vi "单IP测试.vi"(0 "服务端地址":string, 1 "远程端口/服务名称":u16, 3 "本地端口":u16, 8 "连接设置":bool, 11 "模拟数组":u16[](array[numeric]), 16 "06记录":string[][](table), 19 "16记录":string[][](table)) -> (9 "本机ip":string, 12 "接收数据":string, 13 "实时数据":string, 14 "03记录（去重）":string[][](table))   [LabVIEW 2019]
panel:
  out "下发报文":string
  out "格式转换-测试":string
  out "寄存器地址":u16
  out "功能码":u8
  out "从机地址":u8
  in  "停止":bool
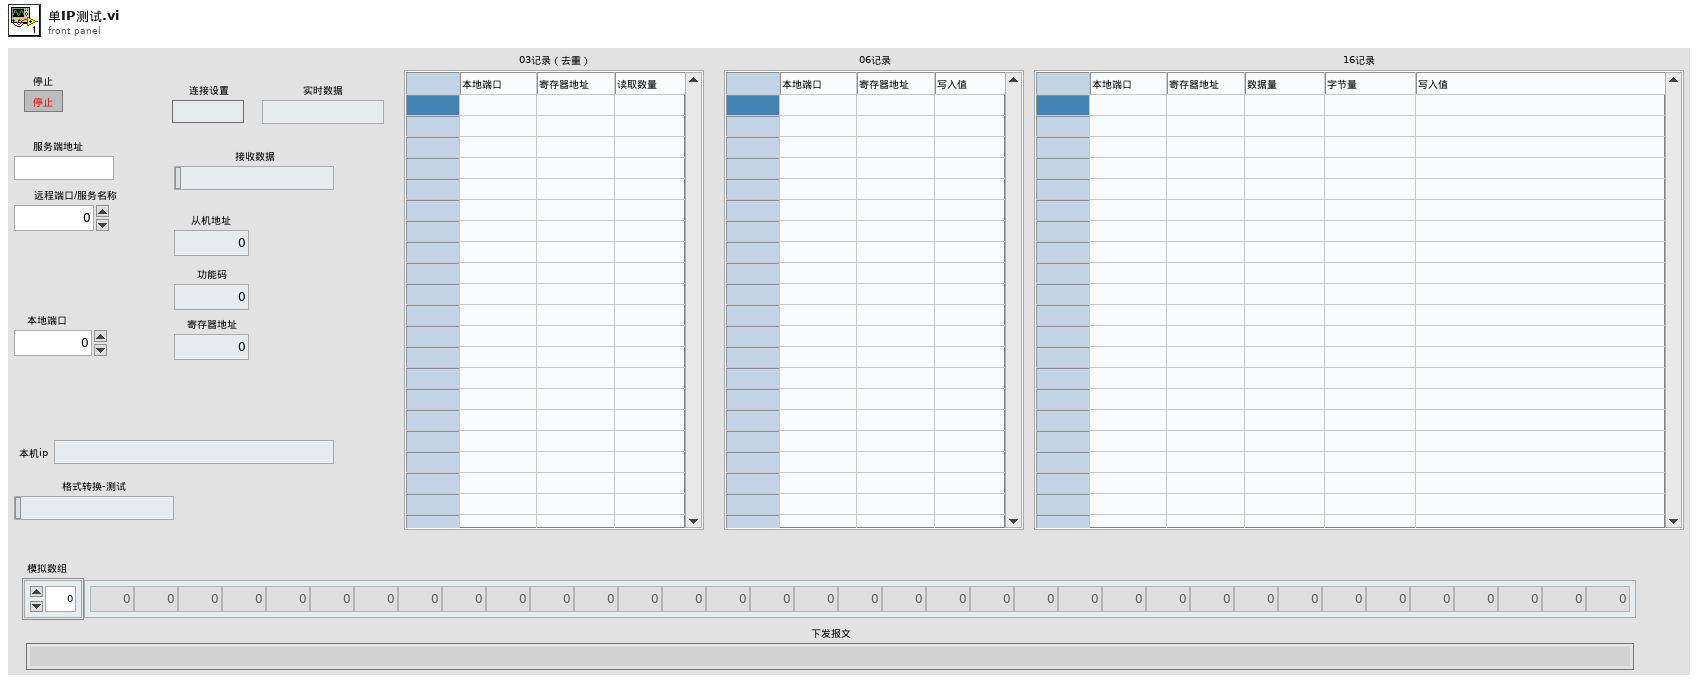
[diagram p1: front panel]
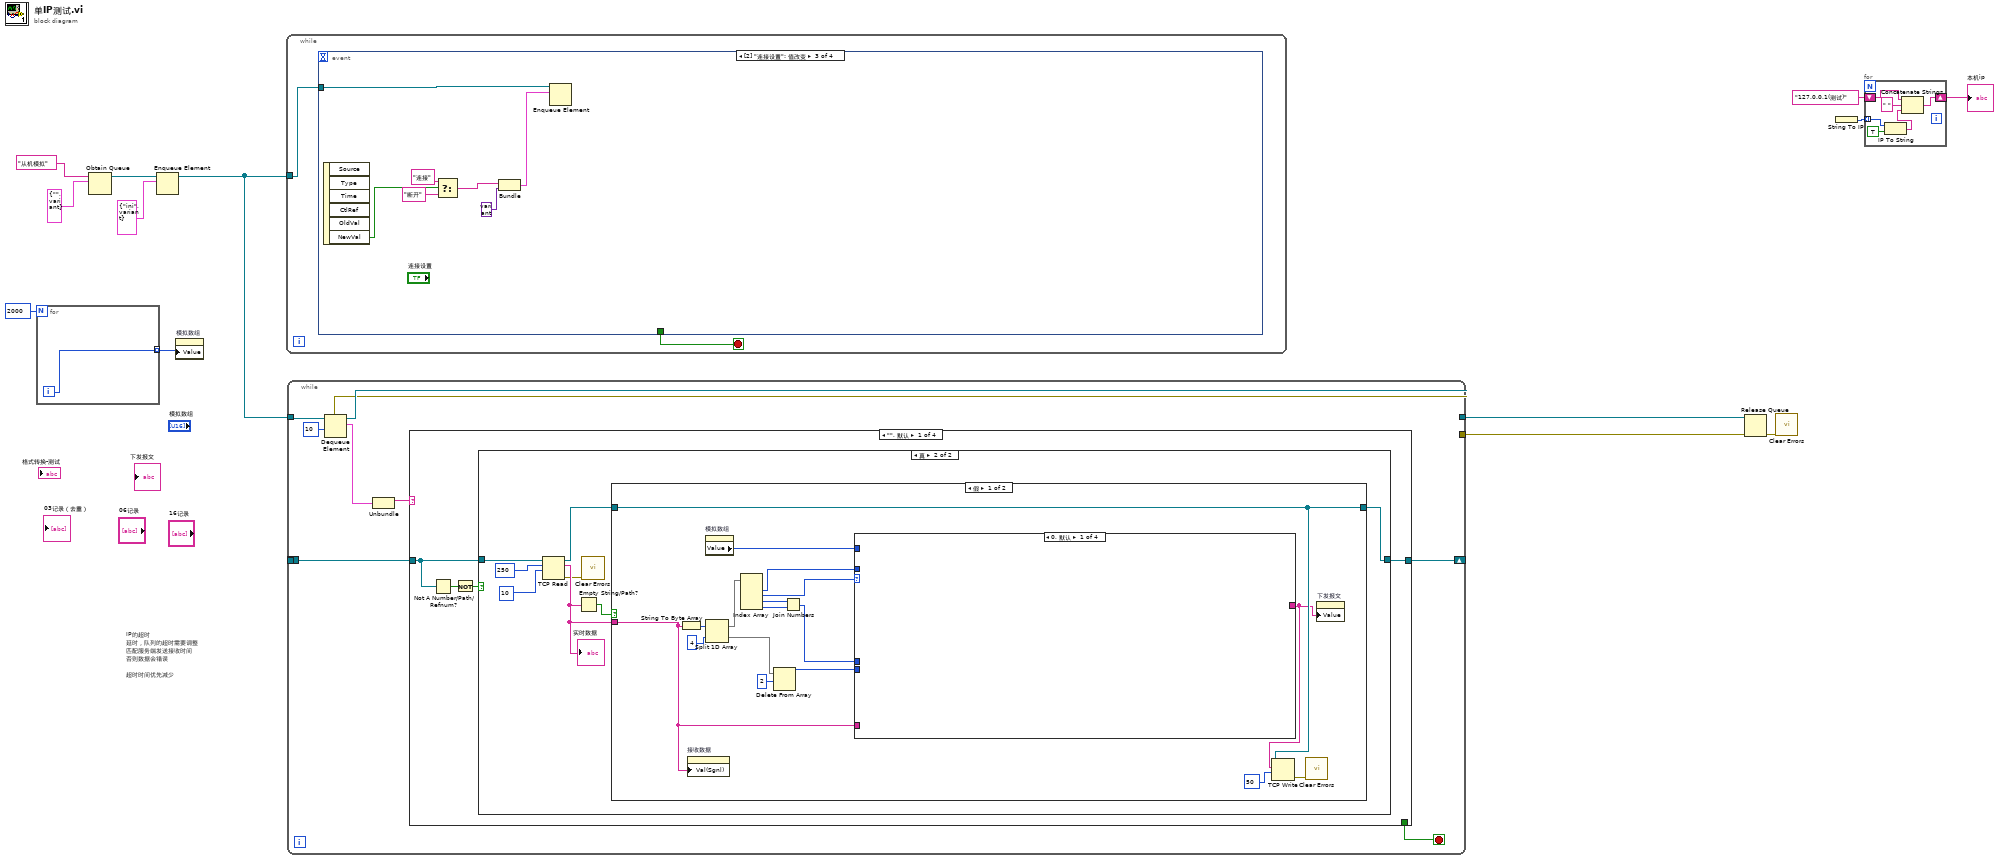
[diagram p0: block diagram]
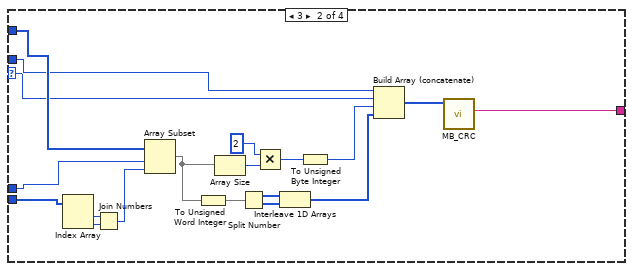
[diagram p3: hidden frame]
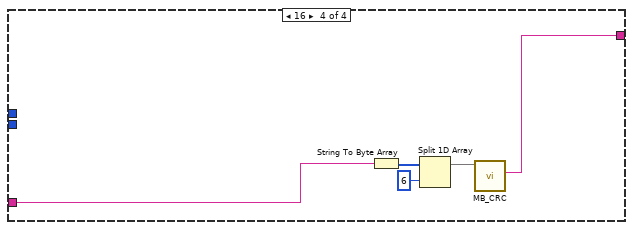
[diagram p5: hidden frame]
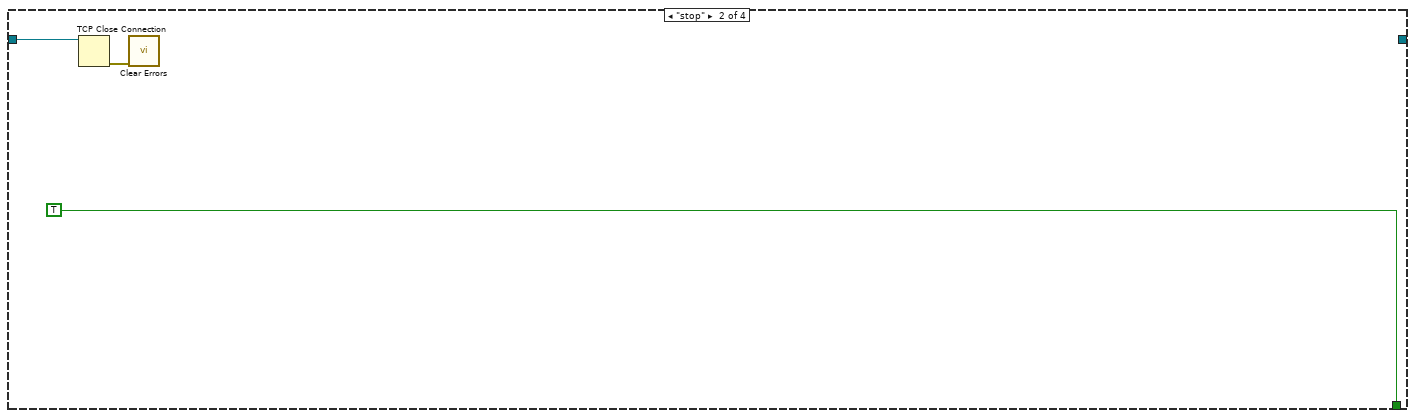
[diagram p7: hidden frame]
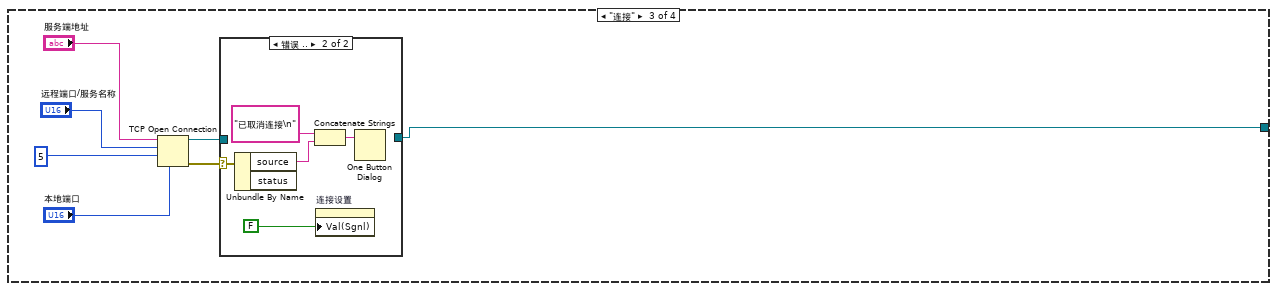
[diagram p8: hidden frame]
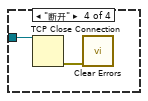
[diagram p10: hidden frame]
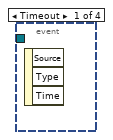
[diagram p11: hidden frame]
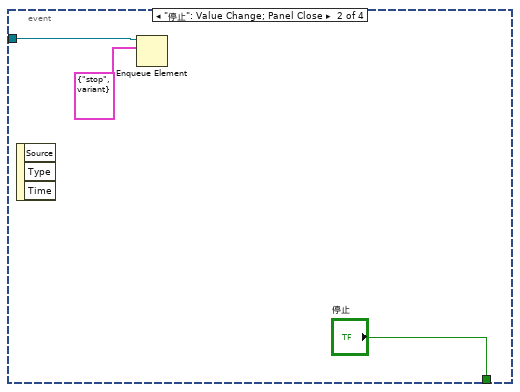
[diagram p12: hidden frame]
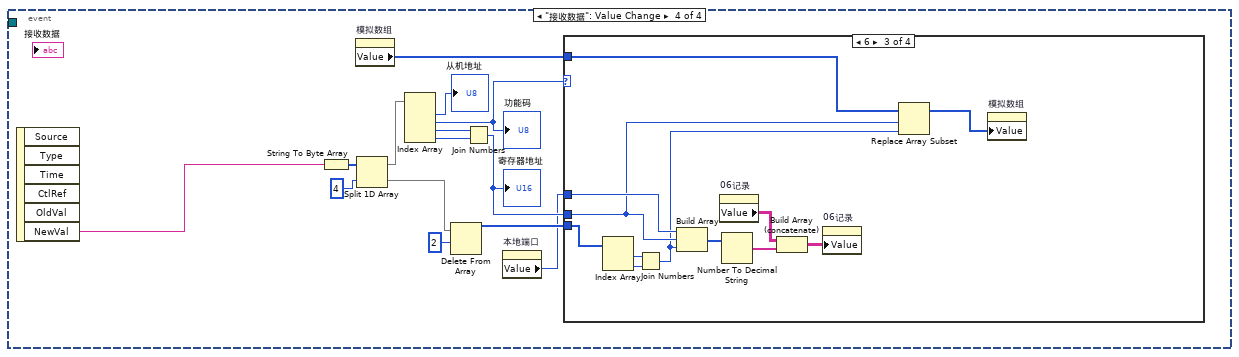
[diagram p13: hidden frame]
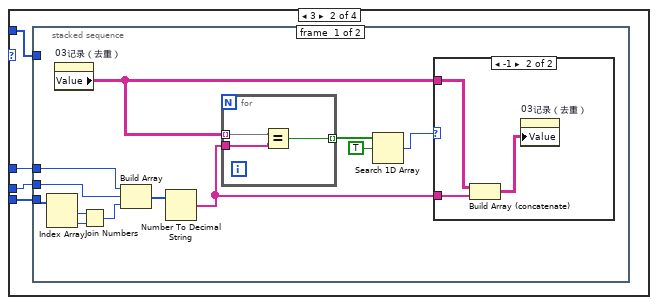
[diagram p15: hidden frame]
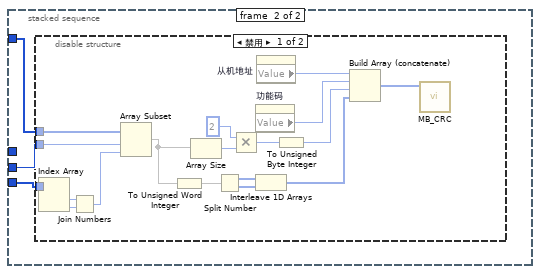
[diagram p17: hidden frame]
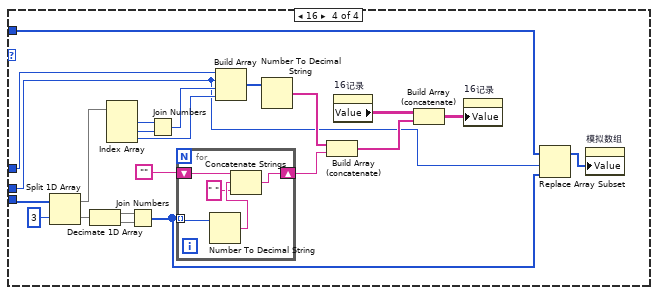
[diagram p19: hidden frame]
diagram:
  # "IP的超时\n延时，队列的超时需要调整\n匹配服务端发送接收时间\n否则数据会错误\n\n超时时间优先减少"
  n1 = for {
    N: 2000 -> [_]
    tunnel: [w14] -> w1 mode=indexing
    i -> [w14]
  }
  n2 = Obtain Queue(name (unnamed)="从机模拟" ("名称（未命名）"), element data type=cluster{string, variant} {"", variant}) -> (queue out=w8:refnum<queue>)  [unwired: 3 in, 2 out]
  n3 = Enqueue Element(queue=w8, element=cluster{string, variant} {"ini", variant} ("元素")) -> (queue out=w6:refnum<queue>)  [unwired: 2 in, 2 out]
  n4 = property on="模拟数组" class="Arr (严格)"("Value"=w1) -> ()  [unwired: 2 in, 2 out]
  n5 = while {
    tunnel: w6 -> [w16]
    stop <- w15 stop-if-true
    n6 = event shown="[2] \"连接设置\": 值改变" {
      selector: _ -> [_ _ _ _]
      dyn-events: _ -> [_ _ _ _]
      timeout: _ -> [_ _ _ _]
      tunnel: [_ "停止" _ _] -> w15
      tunnel: w16 -> [_ w18 w26 _]
      event Timeout {
        n7 = event-data() -> ()  [unwired: 1 in, 3 out]
      }
      event "停止": Value Change; Panel Close {
        n8 = event-data() -> ()  [unwired: 1 in, 3 out]
        n9 = Enqueue Element(queue=w18, element=cluster{string, variant} {"stop", variant} ("元素")) -> ()  [unwired: 2 in, 3 out]
      }
      event "连接设置": Value Change {
        n10 = event-data() -> ("NewVal"=w25:bool)  [unwired: 1 in, 5 out]
        n11 = Select(t="连接", s=w25, f="断开") -> (s? t:f=w23:string)
        n12 = Bundle("f"=w23, variant) -> (w22:cluster{"f":string, variant})  [unwired: 1 in]
        n13 = Enqueue Element(queue=w26, element=w22) -> ()  [unwired: 2 in, 3 out]
      }
      event "接收数据": Value Change {
        n14 = event-data() -> ("NewVal"=w32:string)  [unwired: 1 in, 5 out]
        n15 = String To Byte Array(string=w32) -> (unsigned byte array=w35:u8[])
        n16 = property on="模拟数组" class="Arr (严格)"() -> ("Value"=w27:u16[])  [unwired: 2 in, 2 out]
        n17 = Split 1D Array(array=w35, index=4 ("索引")) -> (first subarray=w36:u8[], second subarray=w40:u8[])
        n18 = Index Array(array=w36) -> (element #1=→"从机地址":u8, element #2=w31:u8, element #3=w38:u8, element #4=w39:u8)  [unwired: 4 in]
        "功能码" <- w31
        n19 = Delete From Array(array=w40, length=2 ("长度")) -> (array with subset deleted=w30:u8[])  [unwired: 1 in, 1 out]
        n20 = Join Numbers(hi=w38, lo=w39) -> ((hi.lo)=w29:u16)
        "寄存器地址" <- w29
        n21 = property on="本地端口" class="DigNum (严格)"() -> ("Value"=w28:u16)  [unwired: 2 in, 2 out]
        n22 = case shown="6" w31 {
          tunnel: w30 -> [_ w43 w91 w116]
          tunnel: w29 -> [_ w44 w86 w98]
          tunnel: w28 -> [_ w42 w90 w117]
          tunnel: w27 -> [_ w41 w87 w99]
          frame 0, Default {
          }
          frame 3 {
            n23 = stacked-sequence {
              tunnel: w44 -> [w56 w64]
              tunnel: w43 -> [w55 w63]
              tunnel: w42 -> [w45 _]
              tunnel: w41 -> [_ w65]
              frame #0 {
                n24 = Index Array(array=w55) -> (element #1=w47:u8, element #2=w48:u8)  [unwired: 2 in]
                n25 = property on="03记录（去重）" class="Tbl (严格)"() -> ("Value"=w49:string[][])  [unwired: 2 in, 2 out]
                n26 = Join Numbers(hi=w47, lo=w48) -> ((hi.lo)=w46:u16)
                n27 = Build Array(w45, w56, w46) -> (w54:u16[])
                n28 = Number To Decimal String(number=w54) -> (decimal integer string=w50:string[])  [unwired: 1 in]
                n29 = for {
                  tunnel: w50 -> [w61]
                  tunnel: w49 -> [w62] mode=indexing
                  tunnel: [w60] -> w53 mode=indexing
                  n30 = Equal?(x=w62, y=w61) -> (x = y?=w60:bool)
                }
                n31 = Search 1D Array(1D array=w53, element=TRUE ("元素")) -> (index of element=w51:i32)  [unwired: 1 in]
                n32 = case shown="-1" w51 {
                  tunnel: w50 -> [_ w59]
                  tunnel: w49 -> [_ w58]
                  frame 0, Default {
                  }
                  frame -1 {
                    n33 = Build Array (concatenate)(w58, w59) -> (w57:string[][])
                    n34 = property on="03记录（去重）" class="Tbl (严格)"("Value"=w57) -> ()  [unwired: 2 in, 2 out]
                  }
                }
              }
              frame #1 {
                n35 = disable-structure shown="禁用" {
                  disable-tunnel: w65 -> [w83 _]
                  disable-tunnel: w64 -> [w82 _]
                  disable-tunnel: w63 -> [w81 _]
                  frame Disabled {
                    n36 = Index Array(array=w81) -> (element #1=w77:u8, element #2=w78:u8)  [unwired: 2 in]
                    n37 = Join Numbers(hi=w77, lo=w78) -> ((hi.lo)=w76:u16)
                    n38 = Array Subset(array=w83, index=w82, length=w76) -> (w70:u16[])
                    n39 = To Unsigned Word Integer(number=w70) -> (unsigned 16bit integer=w69:u16[])
                    n40 = Array Size(array=w70) -> (size(s)=w75:i32)
                    n41 = Split Number(x=w69) -> (hi(x)=w68:u8[], lo(x)=w67:u8[])
                    n42 = Multiply(x=2, y=w75) -> (x*y=w73:i32)
                    n43 = property on="功能码" class="DigNum (严格)"() -> ("Value"=w79:u8)  [unwired: 2 in, 2 out]
                    n44 = Interleave 1D Arrays(w68, w67) -> (w66:u8[])
                    n45 = property on="从机地址" class="DigNum (严格)"() -> ("Value"=w80:u8)  [unwired: 2 in, 2 out]
                    n46 = To Unsigned Byte Integer(number=w73) -> (unsigned 8bit integer=w72:u8)
                    n47 = Build Array (concatenate)(w80, w79, w72, w66) -> (w71:u8[])
                    n48 = call "MB_CRC.vi"("无校验U8数组"=w71) -> ()  [unwired: 6 in, 2 out]
                  }
                  frame Enabled {
                  }
                }
              }
            }
          }
          frame 6 {
            n49 = Index Array(array=w91) -> (element #1=w92:u8, element #2=w93:u8)  [unwired: 2 in]
            n50 = Join Numbers(hi=w92, lo=w93) -> ((hi.lo)=w85:u16)
            n51 = Build Array(w90, w86, w85) -> (w95:u16[])
            n52 = property on="06记录" class="Tbl (严格)"() -> ("Value"=w89:string[][])  [unwired: 2 in, 2 out]
            n53 = Number To Decimal String(number=w95) -> (decimal integer string=w94:string[])  [unwired: 1 in]
            n54 = Build Array (concatenate)(w89, w94) -> (w88:string[][])
            n55 = property on="06记录" class="Tbl (严格)"("Value"=w88) -> ()  [unwired: 2 in, 2 out]
            n56 = Replace Array Subset(array=w87, new element=w85, index=w86) -> (w84:u16[])
            n57 = property on="模拟数组" class="Arr (严格)"("Value"=w84) -> ()  [unwired: 2 in, 2 out]
          }
          frame 16 {
            n58 = Split 1D Array(array=w116, index=3 ("索引")) -> (first subarray=w114:u8[], second subarray=w108:u8[])
            n59 = Decimate 1D Array(w108) -> (w107:u8[], w106:u8[])
            n60 = Index Array(array=w114) -> (element #1=w113:u8, element #2=w112:u8, element #3=w110:u8)  [unwired: 3 in]
            n61 = Join Numbers(hi=w107, lo=w106) -> ((hi.lo)=w97:u16[])
            n62 = Join Numbers(hi=w113, lo=w112) -> ((hi.lo)=w111:u16)
            n63 = for {
              tunnel: w97 -> [w122] mode=indexing
              shift-right: [w119] -> w103
              shift-left: "" -> [w118]
              n64 = Number To Decimal String(number=w122) -> (decimal integer string=w121:string)  [unwired: 1 in]
              n65 = Concatenate Strings(w118, w121, " " ("字符串")) -> (w119:string)
            }
            n66 = Build Array(w117, w98, w111, w110) -> (w109:u16[])
            n67 = Number To Decimal String(number=w109) -> (decimal integer string=w104:string[])  [unwired: 1 in]
            n68 = Build Array (concatenate)(w104, w103) -> (w101:string[])
            n69 = property on="16记录" class="Tbl (严格)"() -> ("Value"=w102:string[][])  [unwired: 2 in, 2 out]
            n70 = Build Array (concatenate)(w102, w101) -> (w100:string[][])
            n71 = property on="16记录" class="Tbl (严格)"("Value"=w100) -> ()  [unwired: 2 in, 2 out]
            n72 = Replace Array Subset(array=w99, new element=w97, index=w98) -> (w96:u16[])
            n73 = property on="模拟数组" class="Arr (严格)"("Value"=w96) -> ()  [unwired: 2 in, 2 out]
          }
        }
      }
    }
  }
  n74 = while {
    tunnel: w6 -> [w131]
    tunnel: [w128] -> w5
    tunnel: [w125] -> w4
    tunnel: [w123] -> _
    shift-right: [w124] -> _
    shift-left: _ -> [w123]
    stop <- w126 stop-if-true
    n75 = Dequeue Element(queue=w131, timeout in ms (-1)=10 ("超时毫秒(-1)")) -> (queue out=w128:refnum<queue>, element=w129:cluster{string, variant}, error out=w125:errorcluster)  [unwired: 1 in, 1 out]
    n76 = Unbundle(w129) -> (w127:string)  [unwired: 1 out]
    n77 = case shown="\"\", 默认" w127 {
      tunnel: [_ TRUE _ _] -> w126
      tunnel: w123 -> [w133 w188 _ w204]
      tunnel: [w132 _ w192 _] -> w124
      frame "", Default {
        n78 = Not A Number/Path/Refnum?(number/path/refnum=w133) -> (NaN/Path/Refnum?=w134:bool)
        n79 = Not(x=w134) -> (.not. x?=w135:bool)
        n80 = case shown="真" w135 {
          tunnel: w133 -> [w136 w144]
          tunnel: [w136 w137] -> w132
          frame False {
          }
          frame True {
            n81 = TCP Read(connection ID=w144, bytes to read=250 ("读取的字节"), 9:10 ("超时毫秒(25000)")) -> (connection ID out=w138:refnum<k5>, data out=w140:string, error out=w139:errorcluster)  [unwired: 2 in]
            "实时数据" <- w140
            n82 = Empty String/Path?(string/path=w140) -> (empty?=w141:bool)
            n83 = call <vilib>:"Clear Errors.vi"("error in (no error)"=w139) -> ()  [unwired: 5 in, 2 out]
            n84 = case shown="假" w141 {
              tunnel: w140 -> [w147 _]
              tunnel: w138 -> [w148 w187]
              tunnel: [w148 w187] -> w137
              frame False {
                n85 = String To Byte Array(string=w147) -> (unsigned byte array=w155:u8[])
                n86 = property on="接收数据" class="Str"("Val(Sgnl)"=w147) -> ()  [unwired: 2 in, 2 out]
                n87 = property on="模拟数组" class="Arr (严格)"() -> ("Value"=w161:u16[])  [unwired: 2 in, 2 out]
                n88 = Split 1D Array(array=w155, index=4 ("索引")) -> (first subarray=w154:u8[], second subarray=w151:u8[])
                n89 = Index Array(array=w154) -> (element #1=w145:u8, element #2=w158:u8, element #3=w153:u8, element #4=w152:u8)  [unwired: 4 in]
                n90 = Delete From Array(array=w151, length=2 ("长度")) -> (array with subset deleted=w159:u8[])  [unwired: 1 in, 1 out]
                n91 = Join Numbers(hi=w153, lo=w152) -> ((hi.lo)=w160:u16)
                n92 = case shown="0, 默认" w158 {
                  selector: w158 -> [_ w175 _ _]
                  tunnel: w159 -> [_ w179 _ _]
                  tunnel: w160 -> [_ w180 _ _]
                  tunnel: w161 -> [_ w178 _ _]
                  tunnel: [_ w177 w181 w182] -> w146
                  tunnel: w147 -> [_ _ w181 w183]
                  tunnel: w145 -> [_ w176 _ _]
                  frame 0, Default {
                  }
                  frame 3 {
                    n93 = Index Array(array=w179) -> (element #1=w173:u8, element #2=w174:u8)  [unwired: 2 in]
                    n94 = Join Numbers(hi=w173, lo=w174) -> ((hi.lo)=w172:u16)
                    n95 = Array Subset(array=w178, index=w180, length=w172) -> (w166:u16[])
                    n96 = To Unsigned Word Integer(number=w166) -> (unsigned 16bit integer=w165:u16[])
                    n97 = Array Size(array=w166) -> (size(s)=w171:i32)
                    n98 = Split Number(x=w165) -> (hi(x)=w164:u8[], lo(x)=w163:u8[])
                    n99 = Multiply(x=2, y=w171) -> (x*y=w169:i32)
                    n100 = Interleave 1D Arrays(w164, w163) -> (w162:u8[])
                    n101 = To Unsigned Byte Integer(number=w169) -> (unsigned 8bit integer=w168:u8)
                    n102 = Build Array (concatenate)(w176, w175, w168, w162) -> (w167:u8[])
                    n103 = call "MB_CRC.vi"("无校验U8数组"=w167) -> ("下发报文"=w177:string)  [unwired: 6 in, 1 out]
                  }
                  frame 6 {
                  }
                  frame 16 {
                    n104 = String To Byte Array(string=w183) -> (unsigned byte array=w186:u8[])
                    n105 = Split 1D Array(array=w186, index=6 ("索引")) -> (first subarray=w184:u8[])  [unwired: 1 out]
                    n106 = call "MB_CRC.vi"("无校验U8数组"=w184) -> ("下发报文"=w182:string)  [unwired: 6 in, 1 out]
                  }
                }
                n107 = TCP Write(connection ID=w148, data in=w146, 9:50 ("超时毫秒(25000)")) -> (error out=w150:errorcluster)  [unwired: 1 in, 2 out]
                n108 = call <vilib>:"Clear Errors.vi"("error in (no error)"=w150) -> ()  [unwired: 5 in, 2 out]
                n109 = property on="下发报文" class="Str"("Value"=w146) -> ()  [unwired: 2 in, 2 out]
              }
              frame True {
              }
            }
          }
        }
      }
      frame "stop" {
        n110 = TCP Close Connection(connection ID=w188) -> (error out=w189:errorcluster)  [unwired: 2 in, 1 out]
        n111 = call <vilib>:"Clear Errors.vi"("error in (no error)"=w189) -> ()  [unwired: 5 in, 2 out]
      }
      frame "连接" {
        n112 = TCP Open Connection(address="服务端地址", remote port or service name="远程端口/服务名称", timeout ms (60000)=5 ("超时毫秒(60000)"), local port="本地端口") -> (connection ID=w197:refnum<k5>, error out=w196:errorcluster)  [unwired: 1 in]
        n113 = case shown="错误 .." w196 {
          selector: w196 -> [_ w203]
          tunnel: [w198 _] -> w192
          tunnel: w197 -> [w198 _]
          frame No Error {
          }
          frame Error {
            n114 = Unbundle By Name(w203) -> ("source"=w201:string)  [unwired: 1 out]
            n115 = Concatenate Strings("已取消连接\n" ("字符串"), w201) -> (w202:string)
            n116 = property on="连接设置" class="Bool (严格)"("Val(Sgnl)"=FALSE ("值(信号)")) -> ()  [unwired: 2 in, 2 out]
            n117 = One Button Dialog(message=w202) -> ()  [unwired: 1 in, 1 out]
          }
        }
      }
      frame "断开" {
        n118 = TCP Close Connection(connection ID=w204) -> (error out=w205:errorcluster)  [unwired: 2 in, 1 out]
        n119 = call <vilib>:"Clear Errors.vi"("error in (no error)"=w205) -> ()  [unwired: 5 in, 2 out]
      }
    }
  }
  n120 = Release Queue(queue=w5, error in (no error)=w4) -> (error out=w3:errorcluster)  [unwired: 1 in, 2 out]
  n121 = call <vilib>:"Clear Errors.vi"("error in (no error)"=w3) -> ()  [unwired: 5 in, 2 out]
  n122 = String To IP() -> (0:w13:u32[])  [unwired: 1 in]
  n123 = for {
    tunnel: w13 -> [w210] mode=indexing
    shift-right: [w206] -> w11
    shift-left: "127.0.0.1(测试)" -> [w207]
    n124 = IP To String(1:TRUE ("句点符号？(F)"), 2:w210) -> (0:w209:string)
    n125 = Concatenate Strings(w207, " " ("字符串"), w209) -> (w206:string)
  }
  "本机ip" <- w11
